vi "Main.vi"() -> ()   [LabVIEW 2020, in "GPackTools.lvlib" / "GPackCLI.lvclass"]
uses:
  GPackCLI.lvclass
  GPackCLI.lvclass/GPackCLI.ctl
panel:
  out "Title":string
  out "Log":string
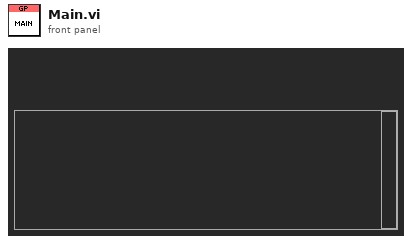
[diagram p1: front panel]
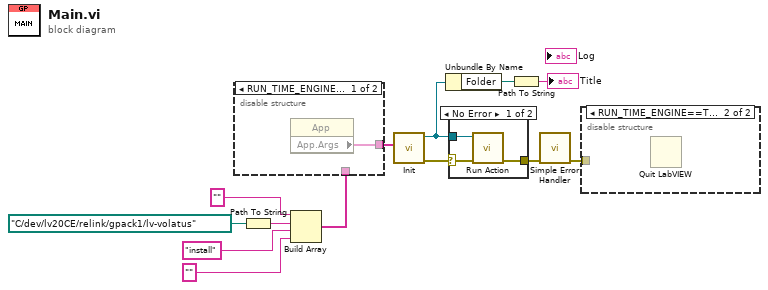
[diagram p0: block diagram]
diagram:
  n1 = Path To String(path=path "C:/dev/lv20CE/relink/gpack1/lv-volatus") -> (string=w7:string)
  n2 = Build Array("", w7, "install", "") -> (w1:string[])
  n3 = disable-structure shown="RUN_TIME_ENGINE==True" {
    disable-tunnel: [w14 w15] -> w2
    disable-tunnel: w1 -> [_ w15]
    frame condition #0 {
      n4 = property class="App"() -> ("App.Args"=w14:string[])  [unwired: 2 in, 2 out]
    }
    frame condition #1 (active) {
    }
  }
  n5 = call "Init.vi"("Args"=w2) -> ("error out"=w4:errorcluster, "GPackCLI out"=w11:refnum<class "GPackCLI.lvclass">)  [unwired: 9 in]
  n6 = Unbundle By Name(w11) -> ("Folder"=w13:path)
  n7 = case shown="No Error" w4 {
    selector: w4 -> [w17 w19]
    tunnel: w11 -> [w18 _]
    tunnel: [w16 w19] -> w10
    frame No Error {
      n8 = call "Run Action.vi"("error in (no error)"=w17, "GPackCLI in"=w18) -> ("error out"=w16:errorcluster)  [unwired: 8 in, 1 out]
    }
    frame Error {
    }
  }
  n9 = Path To String(path=w13) -> (string=→"Title":string)
  n10 = call <vilib>:"Simple Error Handler.vi"("error in (no error)"=w10) -> ("error out"=w9:errorcluster)  [unwired: 4 in, 4 out]
  n11 = disable-structure shown="RUN_TIME_ENGINE==True" {
    disable-tunnel: w9 -> [_ _]
    frame condition #0 (active) {
    }
    frame condition #1 {
      n12 = Quit LabVIEW() -> ()  [unwired: 1 in]
    }
  }
